vi "Set image colour.vi"(11 "Left Image Palette":enum16{"Gray", "Red", "Green"}(ring)) -> (1 "Color Palette":cluster{"Red":u8, "Green":u8, "Blue":u8}[](array[cluster]), 3 "Palette Type":u32)   [LabVIEW 2013]
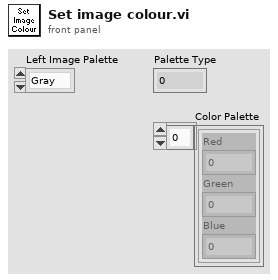
[diagram p1: front panel]
types:
  T1 = enum32{"Gray", "Binary", "Gradient", "Rainbow", "Temperature", "User Defined"}
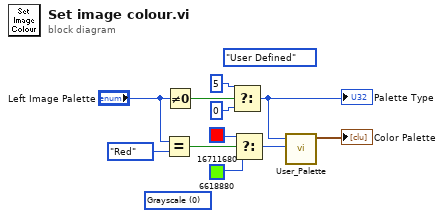
[diagram p0: block diagram]
diagram:
  (unwired) u32 0 items=["Grayscale", "Binary", "Gradient", "Rainbow", "Temperature", "User Defined"] ("Palette:Palette Type")
  (unwired) T1."User Defined" ("Palette Number (gray)")
  n1 = Equal?(x="Left Image Palette", y=enum16{"Gray", "Red", "Green"}."Red") -> (x = y?=w6:bool)
  n2 = Not Equal To 0?(x="Left Image Palette") -> (x != 0?=w1:bool)
  n3 = Select(t=u32 5, s=w1, f=u32 0) -> (s? t:f=w9:u32)
  "Palette Type" <- w9
  n4 = Select(t=u32 16711680 ("Color"), s=w6, f=u32 6618880 ("Color")) -> (s? t:f=w10:u32)
  n5 = call "User_Palette.vi"("Color"=w10, "Palette Number (gray)"=w9) -> ("Color Palette"=→"Color Palette":cluster{"Red":u8, "Green":u8, "Blue":u8}[])  [unwired: 9 in]
